vi "ThridPlatX.vi"(8 "错误输入（无错误）":errorcluster, 10 "CurrentX引用":refnum<vi>, 11 "X引用":refnum<vi>) -> (0 "错误输出":errorcluster, 1 "Direction":i32, 2 "Step":i32, 3 "MotorNum":i32=5)   [LabVIEW 2011]
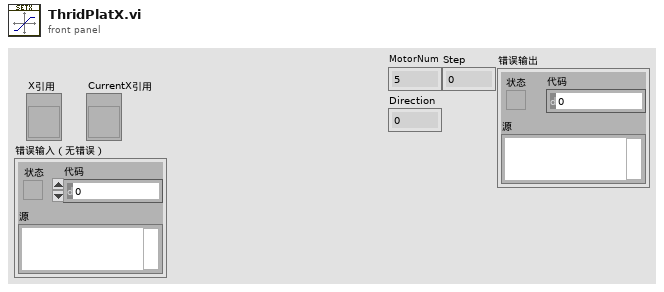
[diagram p1: front panel]
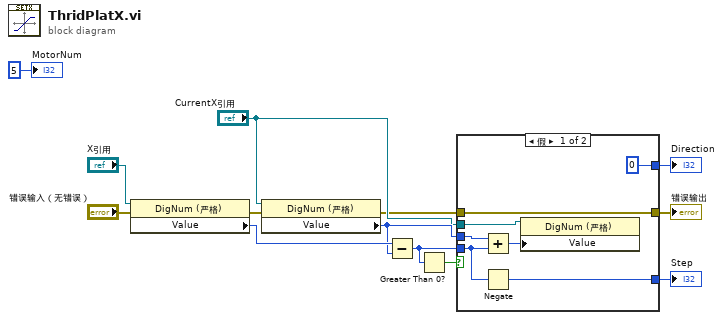
[diagram p0: block diagram]
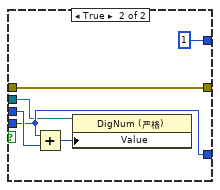
[diagram p2: hidden frame]
diagram:
  n1 = property on="属性节点" class="DigNum (严格)"(reference="X引用", error in="错误输入（无错误）") -> (error out=w4:errorcluster, "Value"=w11:i32)  [unwired: 1 out]
  n2 = property on="属性节点" class="DigNum (严格)"(reference="CurrentX引用", error in=w4) -> (error out=w3:errorcluster, "Value"=w10:i32)  [unwired: 1 out]
  n3 = Subtract(x=w11, y=w10) -> (x-y=w1:i32)
  n4 = Greater Than 0?(x=w1) -> (x > 0?=w13:bool)
  n5 = case shown="假" w13 {
    tunnel: [w19 w24] -> w6
    tunnel: w1 -> [w14 w24]
    tunnel: [0 1] -> w7
    tunnel: w10 -> [w20 w25]
    tunnel: "CurrentX引用" -> [w18 w23]
    tunnel: w3 -> [w15 w21]
    tunnel: [w15 w21] -> w2
    frame False {
      n6 = Add(x=w20, y=w14) -> (x+y=w17:i32)
      n7 = Negate(x=w14) -> (-x=w19:i32)
      n8 = property class="DigNum (严格)"(reference=w18, "Value"=w17) -> ()  [unwired: 1 in, 2 out]
    }
    frame True {
      n9 = Add(x=w24, y=w25) -> (x+y=w22:i32)
      n10 = property class="DigNum (严格)"(reference=w23, "Value"=w22) -> ()  [unwired: 1 in, 2 out]
    }
  }
  "Direction" <- w7
  "Step" <- w6
  "错误输出" <- w2
  "MotorNum" <- 5
